vi "LcArray_Join_STR.vi"(6 "separator":string=",", 8 "error in (no error)":errorcluster, 9 "Array":string[](array[string])) -> (0 "error out":errorcluster, 1 "joined string":string)   [LabVIEW 2019]
doc: "Joins all elements of the input array into a single string. The elements are separated by the separator input."
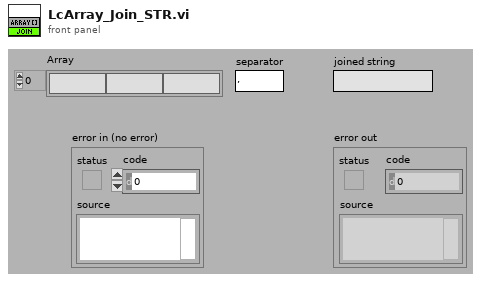
[diagram p1: front panel]
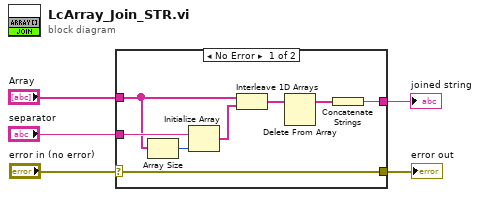
[diagram p0: block diagram]
diagram:
  n1 = case shown="No Error" "error in (no error)" {
    selector: "error in (no error)" -> [w9 w14]
    tunnel: [w8 _] -> w1
    tunnel: "Array" -> [w6 _]
    tunnel: [w9 w14] -> w2
    tunnel: "separator" -> [w7 _]
    frame No Error {
      n2 = Array Size(array=w6) -> (size(s)=w10:i32)
      n3 = Initialize Array(w7, w10) -> (w12:string[])
      n4 = Interleave 1D Arrays(w6, w12) -> (w11:string[])
      n5 = Delete From Array(array=w11) -> (array with subset deleted=w13:string[])  [unwired: 2 in, 1 out]
      n6 = Concatenate Strings(w13) -> (w8:string)
    }
    frame Error {
    }
  }
  "error out" <- w2
  "joined string" <- w1
